vi "AlbumAcquire Callback.vi"(4 "Callback input":T1, 5 "Event Data":cluster{"sender":refnum<k24>, "e":refnum<k24>}, 6 "Control Ref":refnum<k24>, 7 "Event Common Data":T3) -> ()   [LabVIEW 2020]
uses:
  D:/Daguan/Development/RM21-MMicrosopeSource/HardwareAdapter/Camera/Dependencies/PVCamNET.dll
  HardwareAdapter/Camera/Dependencies/PVCamNET.dll
  Callback Input.ctl
  <vilib>/vision/Image Controls.llb/IMAQ Image.ctl
  controls/Image MatadataCtl.ctl
  Global.vi
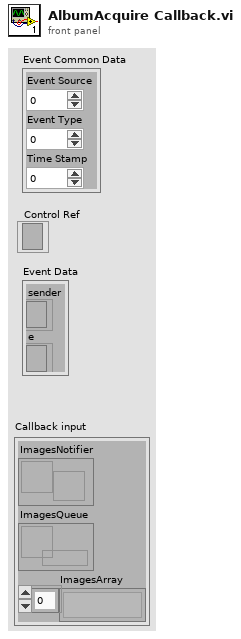
[diagram p1: front panel]
types:
  T1 = typedef "Callback Input.ctl" = cluster{"ImagesNotifier":refnum<notifier>, "ImagesQueue":refnum<queue>, "ImagesArray":T2[]}
  T2 = typedef "IMAQ Image.ctl" = refnum<image>
  T3 = cluster{"Event Source":i32, "Event Type":u32, "Time Stamp":u32}
  T4 = typedef "Image MatadataCtl.ctl" = cluster{"EofTimeStamp(Acq)":dbl, "Image":T2, "Histogram":u32[], "MeanValue":dbl, "Min":u32, "Max":u32, "EofTimeStamp(Album)":dbl, "Fps":dbl, "BufferIndex":u32, "DroppedFrames":u32, "SaveImage?":bool}
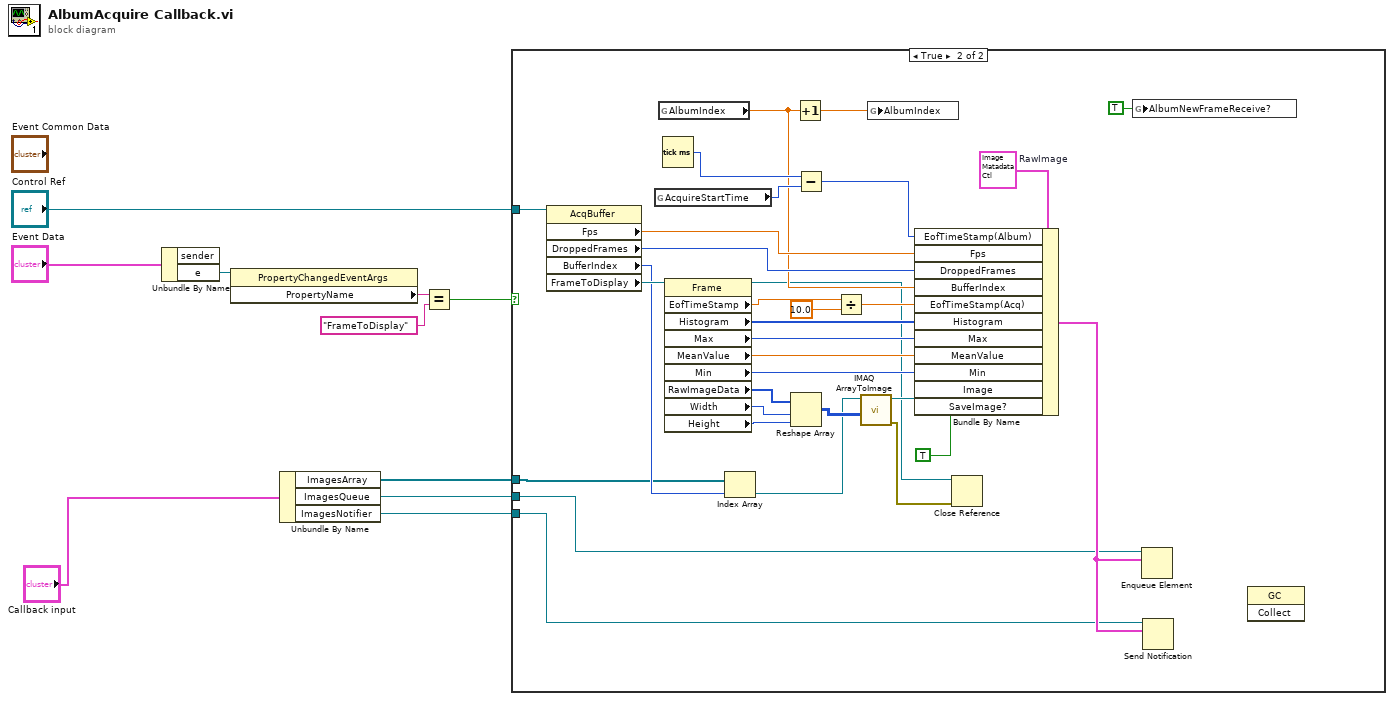
[diagram p0: block diagram]
diagram:
  n1 = Unbundle By Name("Event Data") -> ("e"=w9:refnum<k24>)  [unwired: 1 out]
  n2 = property class="PropertyChangedEventArgs"(reference=w9) -> ("PropertyName"=w8:string)  [unwired: 1 in, 2 out]
  n3 = Unbundle By Name("Callback input") -> ("ImagesArray"=w4:T2[], "ImagesQueue"=w3:refnum<queue>, "ImagesNotifier"=w2:refnum<notifier>)
  n4 = Equal?(x=w8, y="FrameToDisplay") -> (x = y?=w6:bool)
  n5 = case shown="True" w6 {
    tunnel: "Control Ref" -> [_ w42]
    tunnel: w4 -> [_ w24]
    tunnel: w3 -> [_ w11]
    tunnel: w2 -> [_ w12]
    frame False {
    }
    frame True {
      w31 = T4 {"EofTimeStamp(Acq)"=0.0, "Image"=refnum, "Histogram"=[], "MeanValue"=0.0, "Min"=0, "Max"=0, "EofTimeStamp(Album)"=0.0, "Fps"=0.0, "BufferIndex"=0, "DroppedFrames"=0, "SaveImage?"=FALSE}  # RawImage
      n6 = property class="AcqBuffer"(reference=w42) -> ("Fps"=w27:sgl, "DroppedFrames"=w26:i32, "BufferIndex"=w25:i32, "FrameToDisplay"=w41:refnum<k24>)  [unwired: 1 in, 2 out]
      n7 = global read "Global.vi" "AcquireStartTime"() -> (w21:u32)
      n8 = global read "Global.vi" "AlbumIndex"() -> (w17:dbl)
      n9 = Tick Count (ms)() -> (millisecond timer value=w20:u32)
      n10 = property class="Frame"(reference=w41) -> (reference out=w16:refnum<k24>, "EofTimeStamp"=w28:dbl, "Histogram"=w32:u32[], "Max"=w33:u32, "MeanValue"=w34:dbl, "Min"=w37:u32, "RawImageData"=w38:i16[], "Width"=w40:u32, "Height"=w39:u32)  [unwired: 1 in, 1 out]
      n11 = Index Array(array=w24, index=w25) -> (element=w23:T2)
      n12 = Reshape Array "Reshape Array"(w38, w40, w39) -> (w36:i16[][])
      n13 = Increment(x=w17) -> (x+1=w18:dbl)
      n14 = Subtract(x=w20, y=w21) -> (x-y=w19:u32)
      n15 = Divide(x=w28, y=10.0) -> (x/y=w29:dbl)
      n16 = call "IMAQ ArrayToImage"("Image Pixels (I16)"=w36, "Image"=w23) -> ("error out"=w15:errorcluster, "Image Out"=w35:T2)  [unwired: 8 in]
      n17 = global write "Global.vi" "AlbumIndex"(w18) -> ()
      n18 = Bundle By Name(cluster=w31, "EofTimeStamp(Album)"=w19, "Fps"=w27, "DroppedFrames"=w26, "BufferIndex"=w17, "EofTimeStamp(Acq)"=w29, "Histogram"=w32, "Max"=w33, "MeanValue"=w34, "Min"=w37, "Image"=w35, "SaveImage?"=TRUE) -> (w22:T4)
      n19 = Close Reference(reference=w16, error in (no error)=w15) -> ()  [unwired: 1 out]
      n20 = global write "Global.vi" "AlbumNewFrameReceive?"(TRUE ("AlbumNewFrameReceive?")) -> ()
      n21 = Enqueue Element(queue=w11, element=w22) -> ()  [unwired: 2 in, 3 out]
      n22 = Send Notification(notification=w22, notifier=w12) -> ()  [unwired: 1 in, 2 out]
      n23 = invoke class="GC" method="Collect"() -> ()  [unwired: 3 in, 3 out]
    }
  }
